vi "CheckDriveStatus.vi"(2 "Channel Properties":T1={"Channel Name"="", "Vel. Default"=5.0, "Acc. Default"=5.0, "Vel. Max"=5.0, "Vel. Min"=5.0, "Acc. Max"=5.0, "Acc. Min"=5.0, "Pulses/unit"=0.0, "Address"=0, "Pulse Offset"=0, "Pos Tolerance"=0.0, "Pulses/rev"=0.0, "Backlash/Eng units"=0.0, "Current Pos"=0.0, "Ch Status"=enum."Active", "Port Name"="", "Axis Transform mode"="", "Metadata Ch Name"="", "Type"=enum."MCode", "De Power Motor"=enum."FALSE", "ConfigString"=""} {"Current Pos" format="%.2f"; "Backlash/Eng units" format="%.2f"; "Pulses/rev" format="%.2f"; "Pos Tolerance" format="%.2f"; "Pulses/unit" format="%.2f"; "Acc. Min" format="%.2f"; "Acc. Max" format="%.2f"; "Vel. Min" format="%.2f"; "Vel. Max" format="%.2f"; "Acc. Default" format="%.2f"; "Vel. Default" format="%.2f"}, 3 "Axis info cluster":T3) -> (0 "Error string":string, 1 "Axis info cluster Out":T3)   [LabVIEW 2022 SP3]
uses:
  DriveStatus.ctl
  DriveProperties.ctl
  Traverse Type.ctl
  GenericDriveCommand.ctl
  ADAM Client/Sub VIs/ADAM Controls/Remember_value_mode.ctl
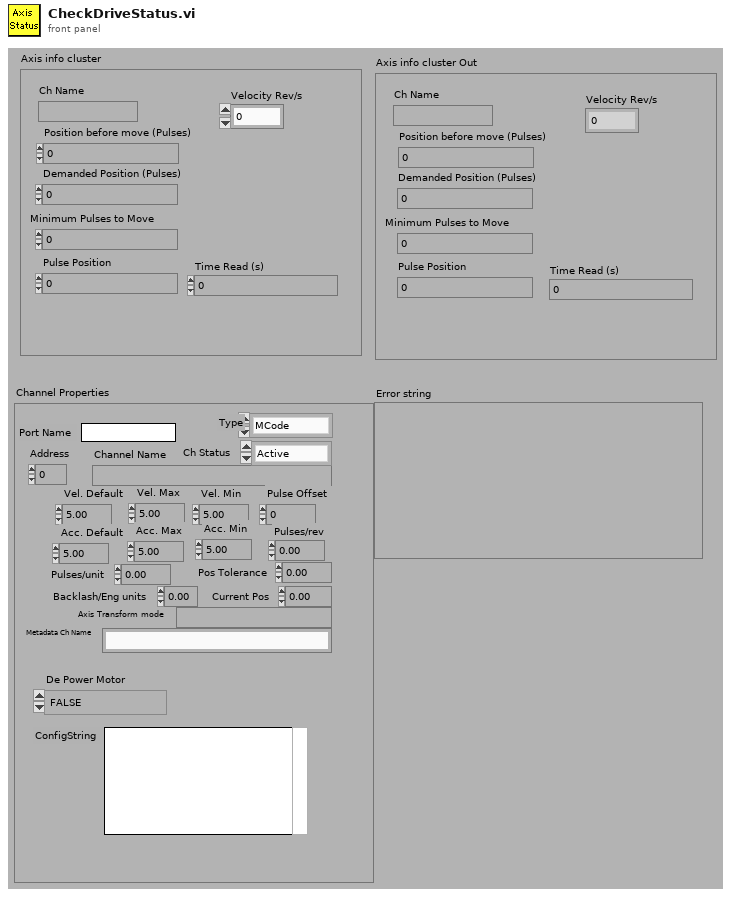
[diagram p1: front panel]
types:
  T1 = typedef "DriveProperties.ctl" = cluster{"Channel Name":string, "Vel. Default":sgl, "Acc. Default":sgl, "Vel. Max":sgl, "Vel. Min":sgl, "Acc. Max":sgl, "Acc. Min":sgl, "Pulses/unit":sgl, "Address":u8, "Pulse Offset":i32, "Pos Tolerance":sgl, "Pulses/rev":sgl, "Backlash/Eng units":sgl, "Current Pos":sgl, "Ch Status":enum16{"Active", "Offline", "Simulate"}, "Port Name":string, "Axis Transform mode":string, "Metadata Ch Name":string, "Type":T2, "De Power Motor":enum16{"TRUE", "FALSE"}, "ConfigString":string}
  T2 = typedef "Traverse Type.ctl" = enum16{"MCode", "Dynamixel"}
  T3 = typedef "DriveStatus.ctl" = cluster{"Ch Name":string, "Position before move (Pulses)":dbl, "Demanded Position (Pulses)":dbl, "Minimum Pulses to Move":dbl, "Pulse Position":dbl, "Time Read (s)":dbl, "Velocity Rev/s":dbl}
  T4 = typedef "GenericDriveCommand.ctl" = string
  T5 = typedef "Remember_value_mode.ctl" = enum16{"Read only", "Read and Write"}
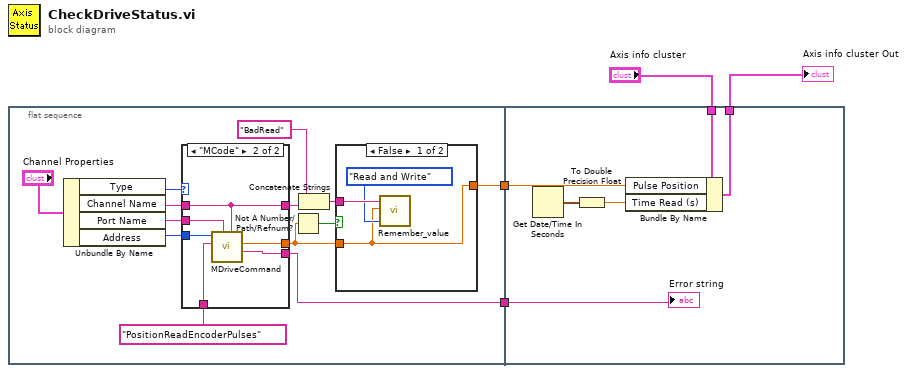
[diagram p0: block diagram]
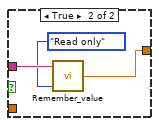
[diagram p2: hidden frame]
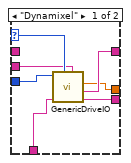
[diagram p3: hidden frame]
diagram:
  n1 = flat-sequence {
    tunnel: [w5] -> w4
    tunnel: [w13] -> w3
    tunnel: w4 -> [w41]
    tunnel: w3 -> [w39]
    tunnel: "Axis info cluster" -> [w42]
    tunnel: [w40] -> w1
    frame #0 {
      n2 = Unbundle By Name("Channel Properties") -> ("Type"=w12:T2, "Channel Name"=w17:string, "Port Name"=w16:string, "Address"=w15:u8)
      n3 = case shown="\"MCode\"" w12 {
        selector: w12 -> [w25 _]
        tunnel: w17 -> [_ w31]
        tunnel: w16 -> [w24 w36]
        tunnel: w15 -> [w30 w35]
        tunnel: [w28 w34] -> w6
        tunnel: [w27 w33] -> w13
        tunnel: T4 "PositionReadEncoderPulses" ("GenericDriveCommand") -> [w26 w32]
        tunnel: [w29 w31] -> w8
        frame "Dynamixel" {
          n4 = call "GenericDriveIO.vi"("GenericDriveCommand"=w26, "Address"=w30, "Type"=w25, "Port Name"=w24) -> ("Error Description"=w27:string, "String Reply"=w29:string, "Numeric Reply"=w28:sgl)  [unwired: 5 in]
        }
        frame "MCode" {
          n5 = call "MDriveCommand.vi"("Channel Name"=w31, "Port Name"=w36, "MDriveCommand"=w32, "Address"=w35) -> ("Error Description"=w33:string, "Numeric Reply"=w34:dbl)  [unwired: 2 in, 3 out]
        }
      }
      n6 = Not A Number/Path/Refnum?(number/path/refnum=w6) -> (NaN/Path/Refnum?=w10:bool)
      n7 = Concatenate Strings("BadRead" ("string"), w8) -> (w7:string)
      n8 = case shown="False" w10 {
        tunnel: w7 -> [w20 w23]
        tunnel: w6 -> [w18 _]
        tunnel: [w18 w21] -> w5
        frame False {
          n9 = call "Remember_value.vi"("Mode"=Remember_value_mode."Read and Write", "Input Value"=w18, "Ch name"=w20) -> ()  [unwired: 1 out]
        }
        frame True {
          n10 = call "Remember_value.vi"("Mode"=Remember_value_mode."Read only", "Ch name"=w23) -> ("Output Value"=w21:dbl)  [unwired: 1 in]
        }
      }
    }
    frame #1 {
      n11 = Get Date/Time In Seconds() -> (seconds since 1Jan1904=w38:timestamp)
      n12 = To Double Precision Float(number=w38) -> (double precision float=w37:dbl)
      n13 = Bundle By Name(cluster=w42, "Pulse Position"=w41, "Time Read (s)"=w37) -> (w40:T3)
      "Error string" <- w39
    }
  }
  "Axis info cluster Out" <- w1
